vi "OE1022D_Configure Frequency.vi"(0 "VISA resource name":refnum<visa-resource-name>, 1 "OE1022D A/B":u8(ring) items=["Channel A", "Channel B"], 2 "Internal Frequency(Hz)":sgl=1000.0 min=0.001 max=100000 step=0.001 format="%.3f", 5 "error in (no error)":errorcluster) -> (14 "VISA resource name out":refnum<visa-resource-name>, 19 "error out":errorcluster)   [LabVIEW 2014]
doc: "Configures the reference source and the internal oscillator."
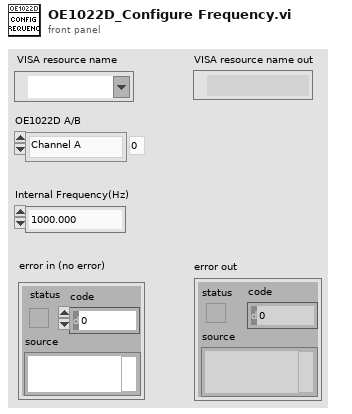
[diagram p1: front panel]
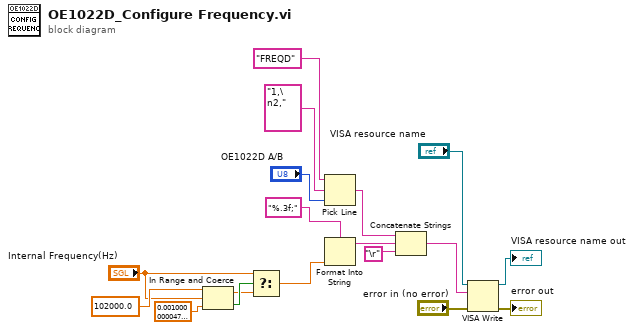
[diagram p0: block diagram]
diagram:
  n1 = In Range and Coerce(upper limit=sgl 102000.0 ("上限"), x="Internal Frequency(Hz)", lower limit=sgl 0.001 ("下限")) -> (coerced(x)=w6:sgl, In Range?=w9:bool)
  n2 = Select(t="Internal Frequency(Hz)", s=w9, f=w6) -> (s? t:f=w11:sgl)
  n3 = Pick Line(string ("")="FREQD", multi-line string="1,\n2,", line index="OE1022D A/B") -> (output string=w4:string)
  n4 = Format Into String(format string="%.3f;", w11) -> (resulting string=w3:string)  [unwired: 2 in, 1 out]
  n5 = Concatenate Strings(w4, w3, "\r") -> (w1:string)
  n6 = VISA Write(VISA resource name="VISA resource name", write buffer=w1, error in (no error)="error in (no error)") -> (VISA resource name out=→"VISA resource name out":refnum<visa-resource-name>, error out=→"error out":errorcluster)  [unwired: 1 out]
